vi "inBound.vi"(1 "j":i32, 2 "i":i32) -> (0 "inBound":bool)   [LabVIEW 2024]
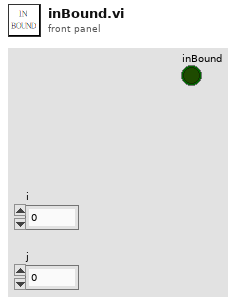
[diagram p1: front panel]
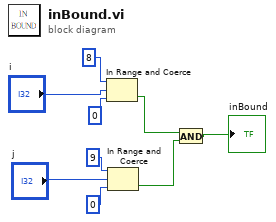
[diagram p0: block diagram]
diagram:
  n1 = In Range and Coerce(upper limit=8, x="i", lower limit=0) -> (In Range?=w3:bool)  [unwired: 1 out]
  n2 = In Range and Coerce(upper limit=9, x="j", lower limit=0) -> (In Range?=w2:bool)  [unwired: 1 out]
  n3 = And(x=w3, y=w2) -> (x .and. y?=→"inBound":bool)
